vi "atan22.vi"(10 "Y":dbl[](array[numeric]), 11 "X":dbl[](array[numeric])) -> (3 "atan2":dbl[](array[numeric]))   [LabVIEW 2011]
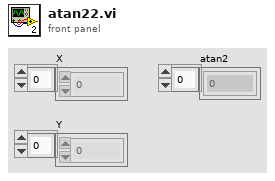
[diagram p1: front panel]
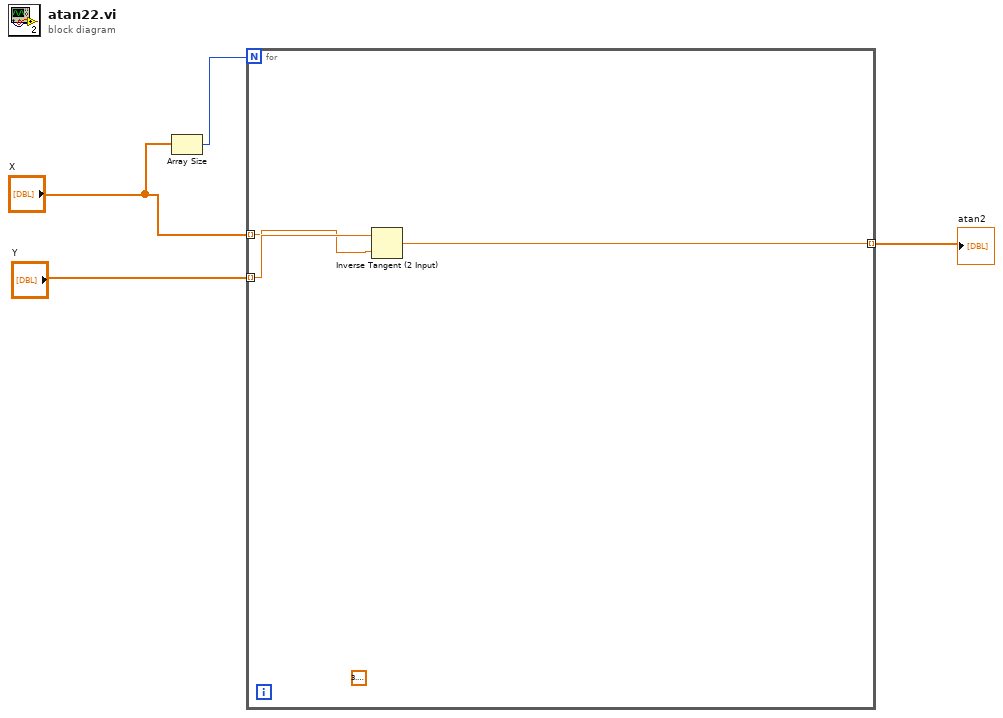
[diagram p0: block diagram]
diagram:
  n1 = Array Size(array="X") -> (size(s)=w3:i32)
  n2 = for {
    N: w3 -> [_]
    tunnel: "Y" -> [w7] mode=indexing
    tunnel: "X" -> [w6] mode=indexing
    tunnel: [w5] -> w1 mode=indexing
    (unwired) 3.141592653589793
    n3 = Inverse Tangent (2 Input)(1:w6, 2:w7) -> (0:w5:dbl)
  }
  "atan2" <- w1
